vi "LRANGE.vi"(0 "refnum in":refnum<vi>, 1 "Key":string, 5 "Start":string, 7 "Stop":string, 11 "error in":errorcluster) -> (4 "refnum out":refnum<vi>, 6 "Data":T1, 15 "error out":errorcluster)   [LabVIEW 2023]
uses:
  SubVIs/Controls/redis-data.ctl
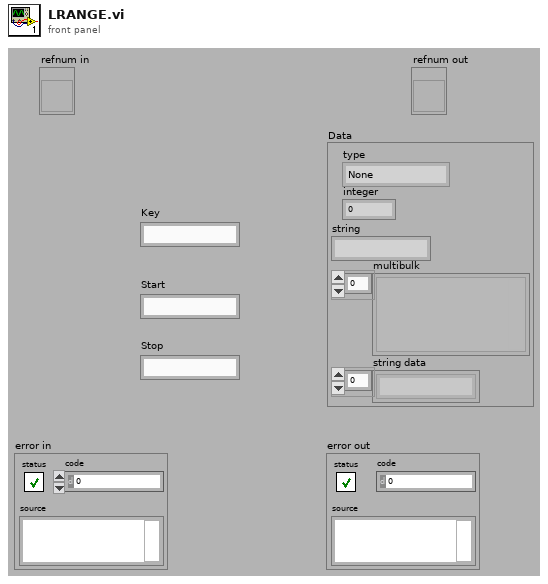
[diagram p1: front panel]
types:
  T1 = typedef "redis-data.ctl" = cluster{"type":enum16{"None", "Error", "Status", "Nil", "Integer", "String", "Multibulk"}, "integer":i64, "string":string, "multibulk":variant[], "string data":string[]}
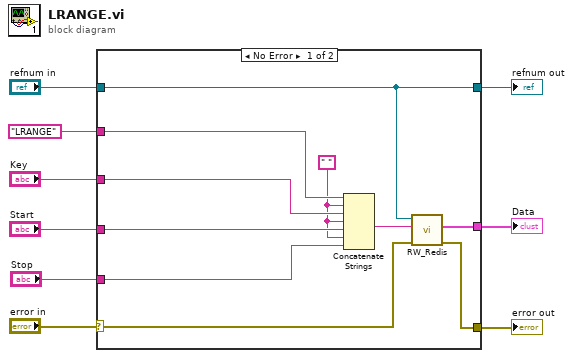
[diagram p0: block diagram]
diagram:
  n1 = case shown="No Error" "error in" {
    selector: "error in" -> [w18 w21]
    tunnel: "LRANGE" -> [w15 _]
    tunnel: "refnum in" -> [w12 w20]
    tunnel: [w17 w21] -> w7
    tunnel: [w16 _] -> w3
    tunnel: "Key" -> [w14 _]
    tunnel: "Start" -> [w13 _]
    tunnel: [w12 w20] -> w2
    tunnel: "Stop" -> [w10 _]
    frame No Error {
      w11 = " "
      n2 = Concatenate Strings(w15, w11, w14, w11, w13, w11, w10) -> (w19:string)
      n3 = call "RW_Redis.vi"("error in"=w18, "command"=w19, "refnum"=w12) -> ("error out"=w17:errorcluster, "Data"=w16:T1)  [unwired: 7 in]
    }
    frame Error {
    }
  }
  "error out" <- w7
  "refnum out" <- w2
  "Data" <- w3
